vi "DashboardShowPopup.vi"(8 "Dashboard":refnum<k24>, 9 "message":string, 11 "error in":errorcluster) -> (0 "Response":cluster{"Message":string, "Succeed":bool}, 3 "error out":errorcluster)   [LabVIEW 2012, in "UnderAutomation.UniversalRobots.lvlib"]
uses:
  UnderAutomation.UniversalRobots.lvlib
  C:/Users/fg/Documents/UniversalRobots.vi/LabVIEW_2024/UnderAutomation.UniversalRobots/lib/UnderAutomation.UniversalRobots.dll
  LabVIEW_2024/UnderAutomation.UniversalRobots/lib/UnderAutomation.UniversalRobots.dll
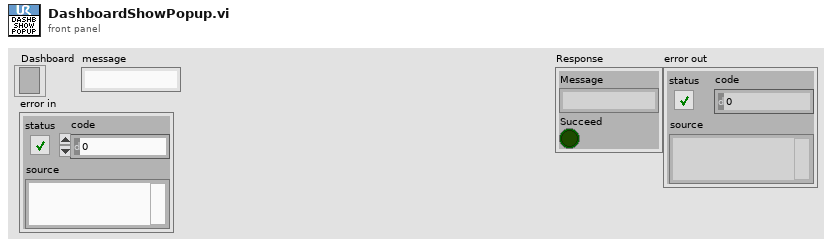
[diagram p1: front panel]
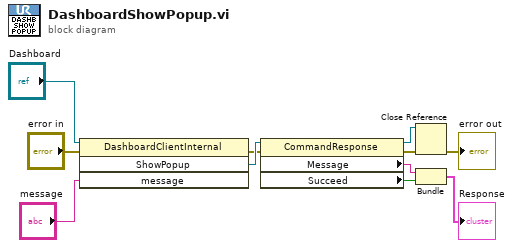
[diagram p0: block diagram]
diagram:
  n1 = invoke class="DashboardClientInternal" method="ShowPopup"(reference="Dashboard", error in="error in", "message"="message") -> (error out=w5:errorcluster, "ShowPopup"=w10:refnum<k24>)  [unwired: 1 in, 2 out]
  n2 = property class="CommandResponse"(reference=w10, error in=w5) -> (reference out=w3:refnum<k24>, error out=w2:errorcluster, "Message"=w9:string, "Succeed"=w8:bool)
  n3 = Close Reference(reference=w3, error in (no error)=w2) -> (error out=→"error out":errorcluster)
  n4 = Bundle("Message"=w9, "Succeed"=w8) -> (→"Response":cluster{"Message":string, "Succeed":bool})  [unwired: 1 in]
